vi "dot frame and fill placement.vi"(6 "Color":u32(colorbox)=16711680, 8 "size":sgl=10.0, 9 "y coordinate":sgl, 10 "x coordinate":sgl, 11 "Image":T1) -> (3 "Image Out":T1)   [LabVIEW 2018]
uses:
  <vilib>/vision/Image Controls.llb/IMAQ Image.ctl
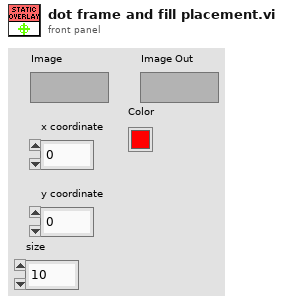
[diagram p1: front panel]
types:
  T1 = typedef "IMAQ Image.ctl" = refnum<image>
  T2 = cluster{"Left":i32, "Top":i32, "Right":i32, "Bottom":i32}
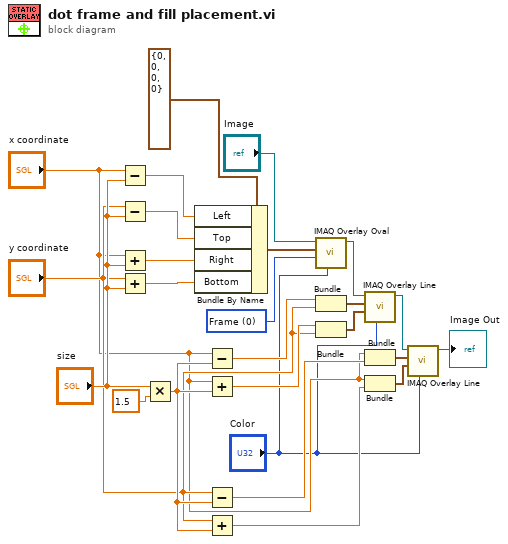
[diagram p0: block diagram]
diagram:
  w19 = u32 0 items=["Frame", "Fill"] ("Drawing Mode (Frame)")
  n1 = Subtract(x="x coordinate", y="size") -> (x-y=w23:sgl)
  n2 = Subtract(x="y coordinate", y="size") -> (x-y=w20:sgl)
  n3 = Add(x="x coordinate", y="size") -> (x+y=w22:sgl)
  n4 = Add(x="y coordinate", y="size") -> (x+y=w21:sgl)
  n5 = Multiply(x="size", y=sgl 1.5) -> (x*y=w13:sgl)
  n6 = Bundle By Name(cluster=T2 {"Left"=0, "Top"=0, "Right"=0, "Bottom"=0} ("Bounding Rectangle"), "Left"=w23, "Top"=w20, "Right"=w22, "Bottom"=w21) -> (w25:T2)
  n7 = Subtract(x="x coordinate", y=w13) -> (x-y=w12:sgl)
  n8 = Add(x="x coordinate", y=w13) -> (x+y=w11:sgl)
  n9 = Subtract(x="y coordinate", y=w13) -> (x-y=w8:sgl)
  n10 = Add(x="y coordinate", y=w13) -> (x+y=w7:sgl)
  n11 = call "IMAQ Overlay Oval"("Color"="Color", "Drawing Mode (Frame)"=w19, "Bounding Rectangle"=w25, "Image"="Image") -> ("Image Out"=w18:T1)  [unwired: 6 in, 1 out]
  n12 = Bundle(w12, "y coordinate"="y coordinate") -> (w17:cluster{sgl, "y coordinate":sgl})  [unwired: 1 in]
  n13 = Bundle(w11, "y coordinate"="y coordinate") -> (w16:cluster{sgl, "y coordinate":sgl})  [unwired: 1 in]
  n14 = call "IMAQ Overlay Line"("Color"="Color", "End Point"=w16, "Start Point"=w17, "Image"=w18) -> ("Image Out"=w4:T1)  [unwired: 6 in, 1 out]
  n15 = Bundle("x coordinate"="x coordinate", w8) -> (w9:cluster{"x coordinate":sgl, sgl})  [unwired: 1 in]
  n16 = Bundle("x coordinate"="x coordinate", w7) -> (w10:cluster{"x coordinate":sgl, sgl})  [unwired: 1 in]
  n17 = call "IMAQ Overlay Line"("Color"="Color", "End Point"=w10, "Start Point"=w9, "Image"=w4) -> ("Image Out"=→"Image Out":T1)  [unwired: 6 in, 1 out]
